vi "4155C Config VAR1 PulsedStressV params.vi"(1 "sweep spacing (linear: 0)":u16(ring) items=["linear", "log 10", "log 25", "log 50"], 6 "step (linear only)":dbl=2.0 format="%^.4e", 7 "sweep mode":u16(ring) items=["Single", "Double"], 8 "error in (no error)":errorcluster, 9 "stop":dbl=10.0 format="%^.4e", 10 "start":dbl format="%^.4e", 11 "VISA session":refnum<visa-resource-name>) -> (0 "error out":errorcluster, 2 "Number of points":i32=1, 3 "dup VISA resource name":refnum<visa-resource-name>)   [LabVIEW 2019]
doc: "This VI configures the primary sweep source (VAR1) for a sweep mode measurement. \n* This VI does not perform error checking on MEASUREMENT MODE or UNIT TYPE of VAR1, therefore it is the application programmer's responsibility to make certain this VI is used in the proper mode."
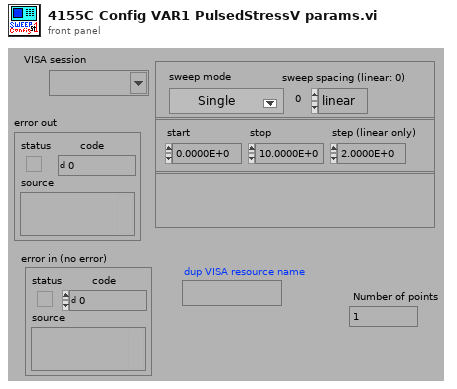
[diagram p1: front panel]
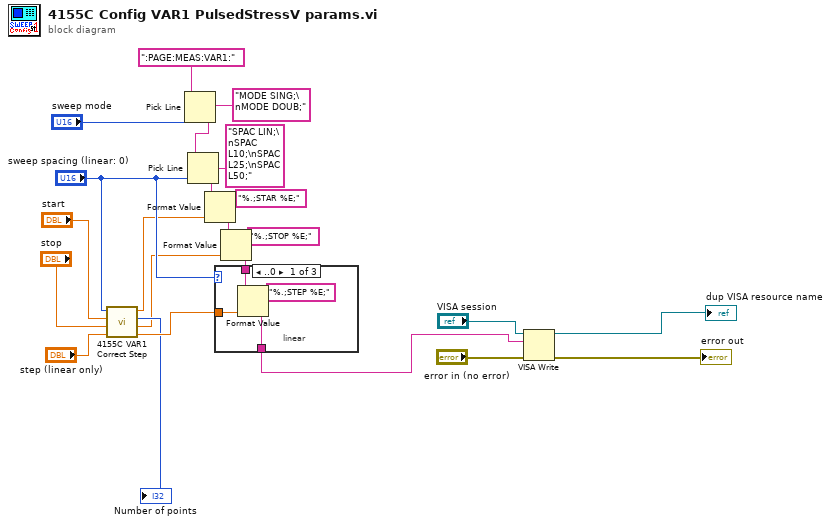
[diagram p0: block diagram]
diagram:
  n1 = call "4155C VAR1 Correct Step.vi"("step"="step (linear only)", "stop"="stop", "start"="start", "sweep spacing (linear: 0)"="sweep spacing (linear: 0)") -> ("Corrected Step"=w7:dbl, "Corrected Stop"=w4:dbl, "Number of points"=→"Number of points":i32, "dup start"=w5:dbl)  [unwired: 4 in]
  n2 = Pick Line(string ("")=":PAGE:MEAS:VAR1:", multi-line string="MODE SING;\nMODE DOUB;", line index="sweep mode") -> (output string=w14:string)
  n3 = Pick Line(string ("")=w14, multi-line string="SPAC LIN;\nSPAC L10;\nSPAC L25;\nSPAC L50;", line index="sweep spacing (linear: 0)") -> (output string=w16:string)
  n4 = Format Value(string ("")=w16, format string="%.;STAR %E;", value (0)=w5) -> (output string=w21:string)
  n5 = Format Value(string ("")=w21, format string="%.;STOP %E;", value (0)=w4) -> (output string=w20:string)
  n6 = case shown="..0" "sweep spacing (linear: 0)" {
    tunnel: w20 -> [w26 w28 w29]
    tunnel: [w25 w28 w29] -> w1
    tunnel: w7 -> [w24 _ _]
    frame ..0 {
      # "linear"
      n7 = Format Value(string ("")=w26, format string="%.;STEP %E;", value (0)=w24) -> (output string=w25:string)
    }
    frame 1 {
      # "log"
    }
    frame 2.. {
      # "log"
    }
  }
  n8 = VISA Write(VISA resource name="VISA session", write buffer=w1, error in (no error)="error in (no error)") -> (VISA resource name out=→"dup VISA resource name":refnum<visa-resource-name>, error out=→"error out":errorcluster)  [unwired: 1 out]
